vi "Sort 2D String Array - Post-process.vi"(0 "Sorted Array (Cols in Original Order. Header row removed)":T1, 1 "Sorted Array (Cols in Sort Order. Header row removed)":T2, 2 "Sorted Array (Cols in Sort Order. Headers as last row)":T3, 4 "Input Array Contains Header Row? (T)":T5, 5 "Sort Ascending? (T)":T4) -> (14 "Column Headers (In Sort Order)":string[](array[string]), 16 "Sorted Data (Columns in Sort Order)":string[][](array[string]), 19 "Sorted Data (Columns in Original Order)":string[][](array[string]))   [LabVIEW 2009, in "xijk_select_best_filter.lvlib"]
doc: "Sort 2D String Array - Post-process.vi\n\n<B>Description:</B>\n\nThis VI processes the strings in the sorted arry into their original format based on information in the meta tag appended to each string in the array.\n\n<B>Usage:</B>\n\nWire all required inputs.\n\n<B>Inputs:</B>\n\nSorted Array (Cols in Original Order. Header row removed)\n- This is the input array of strings sorted in the order specified by the Column Sort Order input with the columns in the original order and the header row removed.\n\nSorted Array (Cols in Sort Order. Header row removed)\n- This is the input array of strings sorted in the order specified by the Column Sort Order input with the columns in the order specified by the Column Sort Order input and the header row removed.\n\nSorted Array (Cols in Sort Order. Headers as last row)\n- This is the input array of strings sorted in the order specified by the Column Sort Order input with the columns in the order specified by the Column Sort Order input and the header row positioned as the last row of the array.\n\nInput Array Contains Header Row? (T)\n- This input indicates if the input array contains a header row.\n\nSort Ascending (T)\n- This input specifies if an ascending or descending sort is to be performed.\n\n<B>Outputs:</B>\n\nColumn Headers (In Sort Order)\n- This output is an array consisting of the column headers in the order specified by the sort order selected by the user.\n\nSorted Data (Columns in Sort Order)\n- This output is an array consisting of the sorted date output with the columns in the order specified by the sort order selected by the user.\n\nSorted Data (Columns in Original Order)\n- This output is an array consisting of the sorted date output with the columns in their original order.\n\n<B>Developed by:</B>\n\nMark Ridgley\nmark.ridgley@logicpd.com"
uses:
  xijk_select_best_filter.lvlib
  _TypeDefs/TYPE - Sorted Array (Cols in Original Order. Header row removed).ctl
  _TypeDefs/TYPE - Sorted Array (Cols in Sort Order. Header row removed).ctl
  _TypeDefs/TYPE - Sorted Array (Cols in Sort Order. Headers as last row).ctl
  _TypeDefs/TYPE - Input Array Contains Header Row.ctl
  _TypeDefs/TYPE - Sort Ascending.ctl
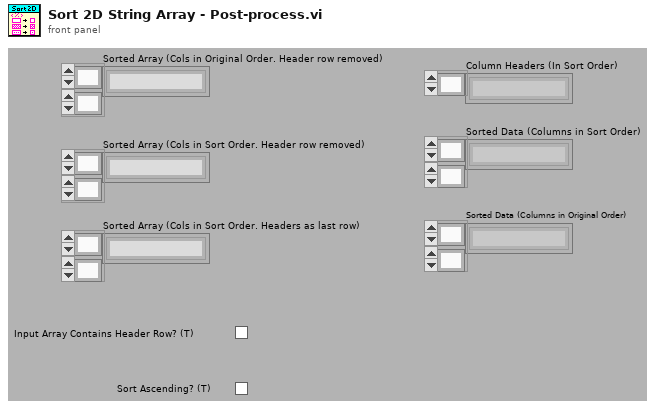
[diagram p1: front panel]
types:
  T1 = typedef "xijk_select_best_filter.lvlib/TYPE - Sorted Array (Cols in Original Order. Header row removed).ctl" = string[][]
  T2 = typedef "xijk_select_best_filter.lvlib/TYPE - Sorted Array (Cols in Sort Order. Header row removed).ctl" = string[][]
  T3 = typedef "xijk_select_best_filter.lvlib/TYPE - Sorted Array (Cols in Sort Order. Headers as last row).ctl" = string[][]
  T4 = typedef "xijk_select_best_filter.lvlib/TYPE - Sort Ascending.ctl" = bool
  T5 = typedef "xijk_select_best_filter.lvlib/TYPE - Input Array Contains Header Row.ctl" = bool
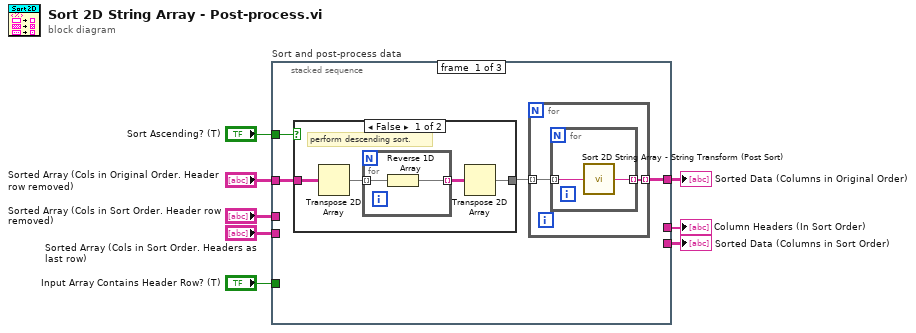
[diagram p0: block diagram]
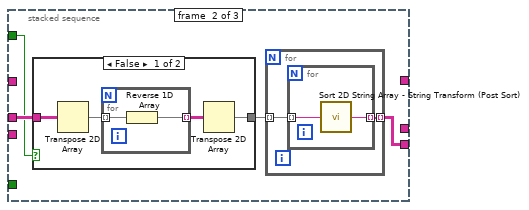
[diagram p3: hidden frame]
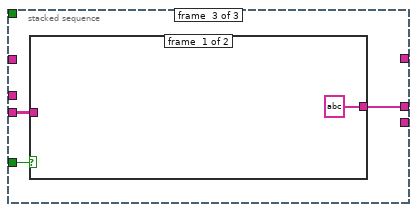
[diagram p5: hidden frame]
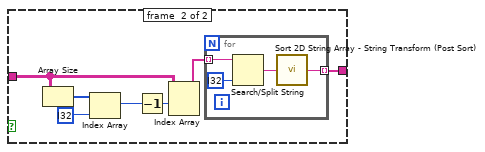
[diagram p6: hidden frame]
diagram:
  n1 = stacked-sequence "Sort and post-process data" {
    tunnel: "Sorted Array (Cols in Original Order. Header row removed)" -> [w11 _ _]
    tunnel: "Sorted Array (Cols in Sort Order. Header row removed)" -> [_ w26 _]
    tunnel: "Sorted Array (Cols in Sort Order. Headers as last row)" -> [_ _ w41]
    tunnel: "Input Array Contains Header Row? (T)" -> [_ _ w40]
    tunnel: "Sort Ascending? (T)" -> [w10 w24 _]
    tunnel: [w9 _ _] -> w6
    tunnel: [_ w25 _] -> w7
    tunnel: [_ _ w39] -> w8
    frame #0 {
      n2 = case shown="False" w10 {
        tunnel: w11 -> [w20 w23]
        tunnel: [w17 w23] -> w12
        frame #0 {
          # "perform descending sort."
          n3 = Transpose 2D Array(2D array=w20) -> (transposed array=w19:T1)
          n4 = for {
            tunnel: w19 -> [w22] mode=indexing
            tunnel: [w21] -> w18 mode=indexing
            n5 = Reverse 1D Array(array=w22) -> (reversed array=w21:string[])
          }
          n6 = Transpose 2D Array(2D array=w18) -> (transposed array=w17:string[][])
        }
        frame #1 {
        }
      }
      n7 = for {
        tunnel: w12 -> [w14] mode=indexing
        tunnel: [w13] -> w9 mode=indexing
        n8 = for {
          tunnel: w14 -> [w16] mode=indexing
          tunnel: [w15] -> w13 mode=indexing
          n9 = call "Sort 2D String Array - String Transform (Post Sort).vi"("Input String (\" \")"=w16) -> ("Output String (\" \")"=w15:string)  [unwired: 14 out]
        }
      }
    }
    frame #1 {
      n10 = case shown="False" w24 {
        tunnel: w26 -> [w35 w38]
        tunnel: [w32 w38] -> w27
        frame #0 {
          n11 = Transpose 2D Array(2D array=w35) -> (transposed array=w34:T2)
          n12 = for {
            tunnel: w34 -> [w37] mode=indexing
            tunnel: [w36] -> w33 mode=indexing
            n13 = Reverse 1D Array(array=w37) -> (reversed array=w36:string[])
          }
          n14 = Transpose 2D Array(2D array=w33) -> (transposed array=w32:string[][])
        }
        frame #1 {
        }
      }
      n15 = for {
        tunnel: w27 -> [w29] mode=indexing
        tunnel: [w28] -> w25 mode=indexing
        n16 = for {
          tunnel: w29 -> [w31] mode=indexing
          tunnel: [w30] -> w28 mode=indexing
          n17 = call "Sort 2D String Array - String Transform (Post Sort).vi"("Input String (\" \")"=w31) -> ("Output String (\" \")"=w30:string)  [unwired: 14 out]
        }
      }
    }
    frame #2 {
      n18 = case shown="True" w40 {
        tunnel: w41 -> [_ w44]
        tunnel: [string[] ? w43] -> w39
        frame #0 {
        }
        frame #1 {
          n19 = Array Size(array=w44) -> (size(s)=w47:i32[])
          n20 = Index Array(array=w47, index=i32 ? ("Index")) -> (element=w45:i32)
          n21 = Decrement(x=w45) -> (x-1=w48:i32)
          n22 = Index Array(array=w44, index (row)=w48) -> (element=w49:string[])  [unwired: 1 in]
          n23 = for {
            tunnel: w49 -> [w53] mode=indexing
            tunnel: [w50] -> w43 mode=indexing
            n24 = Search/Split String(string=w53, offset (0)=i32 ?) -> (match + rest of string=w51:string)  [unwired: 3 out]
            n25 = call "Sort 2D String Array - String Transform (Post Sort).vi"("Input String (\" \")"=w51) -> ("Output String (\" \")"=w50:string)  [unwired: 14 out]
          }
        }
      }
    }
  }
  "Column Headers (In Sort Order)" <- w8
  "Sorted Data (Columns in Sort Order)" <- w7
  "Sorted Data (Columns in Original Order)" <- w6
